vi "Main.vi"() -> ()   [LabVIEW 2015]
uses:
  TypeDefs/Buttons UI.ctl
  TypeDefs/States.ctl
  TypeDefs/Acq Loop Data.ctl
panel:
  in  "#samples":dbl=100.0
  in  "Frequency":dbl=1000.0
  out "File Path":path
  in  "File Name Prefix":string="LV Academy"
  in  "Buttons":T1
  out "Wykres":dbl[](graph)
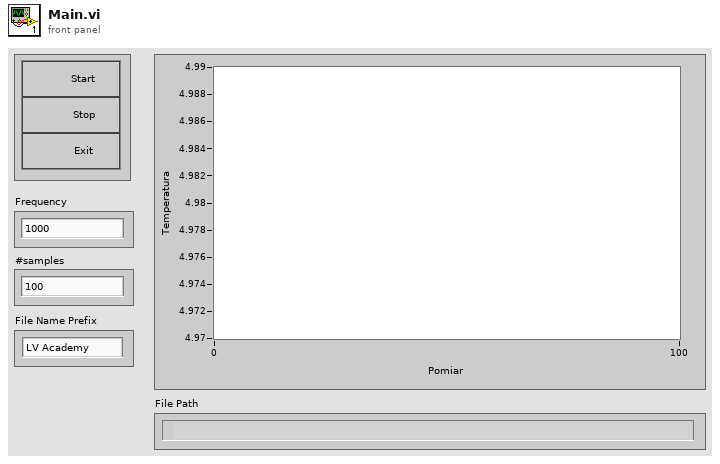
[diagram p1: front panel]
types:
  T1 = typedef "Buttons UI.ctl" = cluster{"Start":bool, "Stop":bool, "Exit":bool}
  T2 = typedef "Acq Loop Data.ctl" = cluster{"File Name Profix":string, "Frequency":dbl, "#samples":i32, "DAQ task ":refnum<k21>}
  T3 = typedef "Queue Data" = cluster{"Action":string, "Data":dbl[]}
  T4 = typedef "States.ctl" = enum16{"Check if Stop or Exit", "Exit", "Wait for Start or Exit", "Start Acquisition", "Reset Acquisition", "Acquisition"}
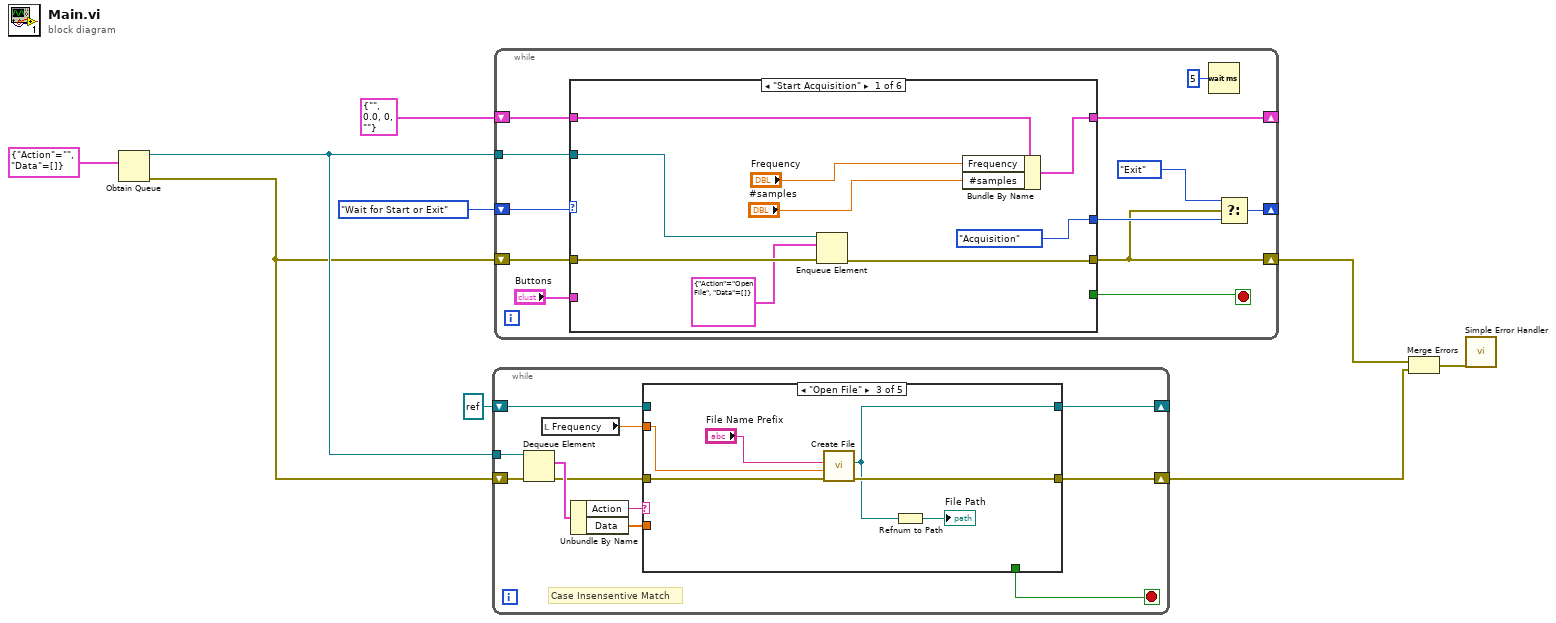
[diagram p0: block diagram]
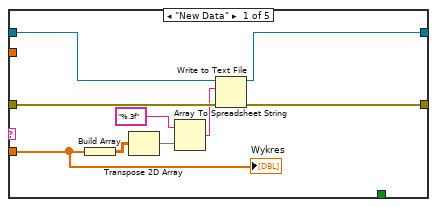
[diagram p2: hidden frame]
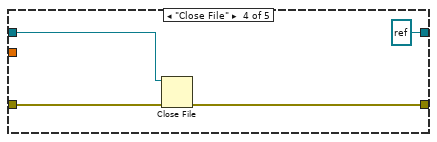
[diagram p4: hidden frame]
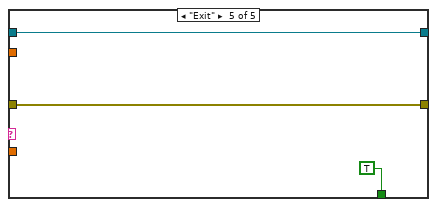
[diagram p5: hidden frame]
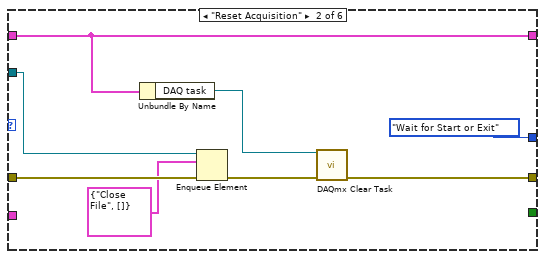
[diagram p6: hidden frame]
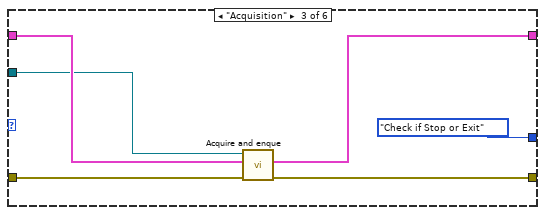
[diagram p7: hidden frame]
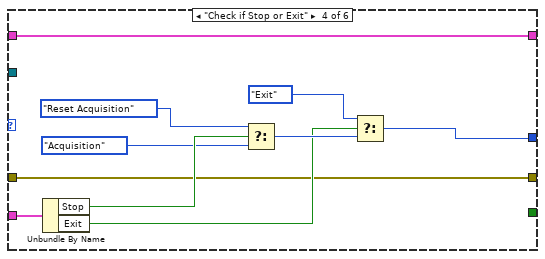
[diagram p8: hidden frame]
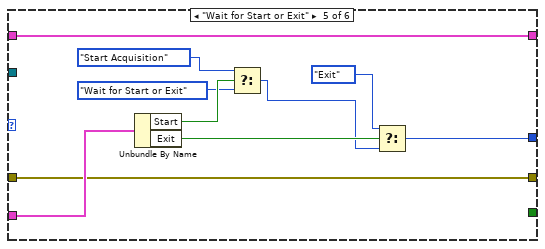
[diagram p9: hidden frame]
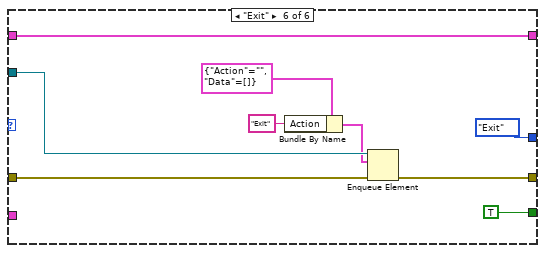
[diagram p10: hidden frame]
diagram:
  n1 = Obtain Queue(element data type=T3 {"Action"="", "Data"=[]}) -> (queue out=w7:refnum<queue>, error out=w6:errorcluster)  [unwired: 4 in, 1 out]
  n2 = while {
    tunnel: w7 -> [w20]
    shift-right: [w13] -> w3
    shift-left: w6 -> [w19]
    shift-right: [w14] -> _
    shift-left: refnum<file> refnum ("refnum out") -> [w12]
    stop <- w11 stop-if-true
    # "Case Insensentive Match"
    n3 = Dequeue Element(queue=w20, error in (no error)=w19) -> (element=w18:T3, error out=w15:errorcluster)  [unwired: 1 in, 2 out]
    n4 = local read "Frequency"() -> (w10:dbl)
    n5 = Unbundle By Name(w18) -> ("Action"=w17:string, "Data"=w16:dbl[])
    n6 = case shown="\"Open File\"" w17 {
      tunnel: w16 -> [w23 _ _ _ _]
      tunnel: w15 -> [w28 w31 w37 w41 w43]
      tunnel: [w25 w30 w33 refnum<file> refnum ("refnum out") w42] -> w14
      tunnel: [w24 w31 w35 w39 w43] -> w13
      tunnel: w12 -> [w26 w30 _ w40 w42]
      tunnel: [_ _ _ _ TRUE] -> w11
      tunnel: w10 -> [_ _ w32 _ _]
      frame "New Data" {
        n7 = Build Array(w23) -> (w21:dbl[][])
        n8 = Transpose 2D Array(2D array=w21) -> (transposed array=w22:dbl[][])
        n9 = Array To Spreadsheet String(array=w22, 3:"%.3f") -> (spreadsheet string=w27:string)  [unwired: 1 in]
        n10 = Write to Text File(file (use dialog)=w26, text=w27, error in=w28) -> (refnum out=w25:refnum<file>, error out=w24:errorcluster)  [unwired: 1 in, 1 out]
        "Wykres" <- w23
      }
      frame Default {
      }
      frame "Open File" {
        n11 = call "Create File.vi"("error in (no error)"=w37, "Numeric"=w32, "Folder Name Prefix"="File Name Prefix") -> ("error out"=w35:errorcluster, "refnum out"=w33:refnum<file>)  [unwired: 7 in]
        n12 = Refnum to Path(1:w33) -> (0:→"File Path":path)
      }
      frame "Close File" {
        n13 = Close File(refnum=w40, error in=w41) -> (error out=w39:errorcluster)  [unwired: 1 out]
      }
      frame "Exit" {
      }
    }
  }
  n14 = while {
    shift-right: [w47] -> _
    shift-left: States."Wait for Start or Exit" -> [w56]
    tunnel: w7 -> [w54]
    shift-right: [w51] -> _
    shift-left: T2 {"File Name Profix"="", "Frequency"=0.0, "#samples"=0, "DAQ task "=""} -> [w52]
    shift-right: [w45] -> w2
    shift-left: w6 -> [w55]
    stop <- w49 stop-if-true
    n15 = case shown="\"Start Acquisition\"" w56 {
      tunnel: w55 -> [w60 w70 w79 w81 w92 w107]
      tunnel: w54 -> [w58 w68 w77 _ _ w105]
      tunnel: "Buttons" -> [_ _ _ w89 w99 _]
      tunnel: [States."Acquisition" States."Wait for Start or Exit" States."Check if Stop or Exit" w82 w94 States."Exit"] -> w48
      tunnel: w52 -> [w65 w66 w78 w80 w93 w101]
      tunnel: [w62 w66 w74 w80 w93 w101] -> w51
      tunnel: [w59 w73 w76 w81 w92 w106] -> w45
      tunnel: [_ _ _ _ _ TRUE] -> w49
      frame "Start Acquisition" {
        n16 = Enqueue Element(queue=w58, element=T3 {"Action"="Open File", "Data"=[]}, error in (no error)=w60) -> (error out=w59:errorcluster)  [unwired: 1 in, 2 out]
        n17 = Bundle By Name(cluster=w65, "Frequency"="Frequency", "#samples"="#samples") -> (w62:T2)
      }
      frame "Reset Acquisition" {
        n18 = Unbundle By Name(w66) -> ("DAQ task"=w72:refnum<k21>)
        n19 = Enqueue Element(queue=w68, element=T3 {"Action"="Close File", "Data"=[]}, error in (no error)=w70) -> (error out=w69:errorcluster)  [unwired: 1 in, 2 out]
        n20 = call <vilib>:"DAQmx Clear Task.vi"("task in"=w72, "error in"=w69) -> ("error out"=w73:errorcluster)  [unwired: 13 in]
      }
      frame "Acquisition" {
        n21 = call "Acquire and enque.vi"("error in (no error)"=w79, "Data In"=w78, "Queue in"=w77) -> ("error out"=w76:errorcluster, "Data Out"=w74:T2)  [unwired: 7 in]
      }
      frame "Check if Stop or Exit" {
        n22 = Unbundle By Name(w89) -> ("Stop"=w88:bool, "Exit"=w84:bool)
        n23 = Select(t=States."Reset Acquisition", s=w88, f=States."Acquisition") -> (s? t:f=w85:T4)
        n24 = Select(t=States."Exit", s=w84, f=w85) -> (s? t:f=w82:T4)
      }
      frame "Wait for Start or Exit" {
        n25 = Unbundle By Name(w99) -> ("Start"=w98:bool, "Exit"=w95:bool)
        n26 = Select(t=States."Start Acquisition", s=w98, f=States."Wait for Start or Exit") -> (s? t:f=w91:T4)
        n27 = Select(t=States."Exit", s=w95, f=w91) -> (s? t:f=w94:T4)
      }
      frame "Exit" {
        n28 = Bundle By Name(cluster=T3 {"Action"="", "Data"=[]}, "Action"="Exit") -> (w102:T3)
        n29 = Enqueue Element(queue=w105, element=w102, error in (no error)=w107) -> (error out=w106:errorcluster)  [unwired: 1 in, 2 out]
      }
    }
    n30 = Wait (ms)(milliseconds to wait=u32 5) -> ()  [unwired: 1 out]
    n31 = Select(t=States."Exit", s=w45, f=w48) -> (s? t:f=w47:T4)
  }
  n32 = Merge Errors(w2, w3) -> (w1:errorcluster)
  n33 = call <vilib>:"Simple Error Handler.vi"("error in (no error)"=w1) -> ()  [unwired: 4 in, 5 out]
